vi "Leap Close.vi"(8 "error in (no error)":errorcluster, 11 "Leap Handle In":T1) -> (0 "error out":errorcluster)   [LabVIEW 2011, in "LVH-Leap.lvlib"]
doc: "Close the Leap Controller Handle to safely clean-up resources used by the API"
uses:
  LVH-Leap.lvlib
  Private/Type Defs/Leap Handle.ctl
  C:/github/labviewhacker/LVH-Leap/LabVIEW/vi.lib/LabVIEW Hacker/Leap/Private/Libs/LeapCSharp.NET3.5.dll
  Private/Libs/LeapCSharp.NET3.5.dll
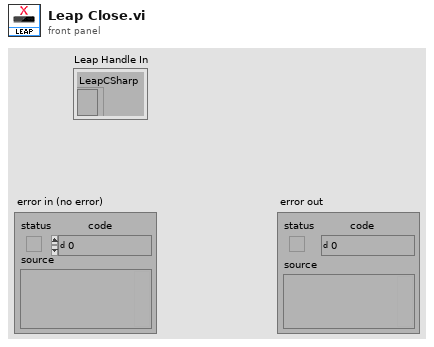
[diagram p1: front panel]
types:
  T1 = typedef "LVH-Leap.lvlib/Leap Handle.ctl" = cluster{"LeapCSharp":refnum<k24>}
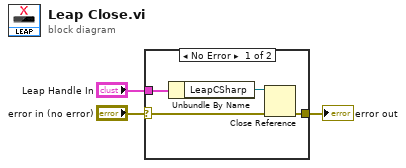
[diagram p0: block diagram]
diagram:
  n1 = case shown="No Error" "error in (no error)" {
    selector: "error in (no error)" -> [w4 w8]
    tunnel: [w6 w8] -> w2
    tunnel: "Leap Handle In" -> [w7 _]
    frame No Error {
      n2 = Unbundle By Name(w7) -> ("LeapCSharp"=w5:refnum<k24>)
      n3 = Close Reference(reference=w5, error in (no error)=w4) -> (error out=w6:errorcluster)
    }
    frame Error {
    }
  }
  "error out" <- w2
